vi "I2C_ID_Check.vi"() -> ()   [LabVIEW 2017]
uses:
  <vilib>/myRIO/Common/Instrument Driver Framework/myRIO v1.0/UART/vis/myRIO v1.0 Close UART.vi
  <vilib>/myRIO/Common/Instrument Driver Framework/Utilities/vis/FPGA Ref Manager.vi
  <vilib>/myRIO/Common/Instrument Driver Framework/myRIO v1.0/myRIO v1.0 Reset FPGA.vi
  <vilib>/myRIO/Common/Instrument Driver Framework/myRIO v1.0/IRQ/vis/myRIO v1.0 IRQ Info FGV.vi
  <vilib>/myRIO/Common/Instrument Driver Framework/myRIO v1.0/IRQ/vis/myRIO v1.0 Timer IRQ Info FGV.vi
  <vilib>/myRIO/Common/Instrument Driver Framework/myRIO v1.0/IRQ/vis/myRIO v1.0 ISR Agent.vi
  <vilib>/myRIO/Instrument Drivers/Utilities/Utilities.lvlib
panel:
  out "Controller ID# Found":u8
  out "error out":errorcluster
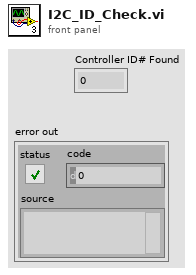
[diagram p1: front panel]
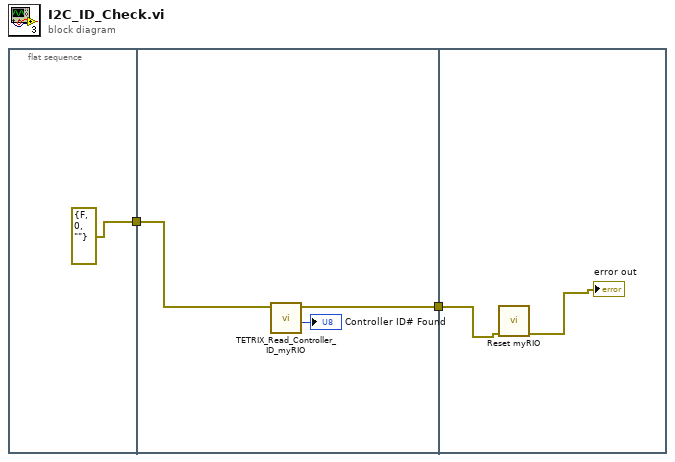
[diagram p0: block diagram]
diagram:
  n1 = flat-sequence {
    tunnel: [errorcluster {"status"=FALSE, "code"=0, "source"=""} ("error constant")] -> w1
    tunnel: [w6] -> w2
    tunnel: w1 -> [w4]
    tunnel: w2 -> [w8]
    frame #0 {
    }
    frame #1 {
      n2 = call <vilib>:"TETRIX_Read_Controller_ID_myRIO.vi"("Error/Flow In"=w4) -> ("Controller ID# Found"=→"Controller ID# Found":u8, "Error/Flow Out"=w6:errorcluster)  [unwired: 5 in]
    }
    frame #2 {
      n3 = call <vilib>:"Reset myRIO.vi"("error in (no error)"=w8) -> ("error out"=→"error out":errorcluster)  [unwired: 10 in]
    }
  }
